vi "Rotate triangle about arbitrary axis.vi"(1 "Rotation angle (rad)":sgl, 2 "Rotation axis coordinates (x, y, z)":sgl[](array[numeric]), 3 "Rotation axis (unit direction vector)\nanti-clockwise positive looking into axis":sgl[](array[numeric]), 4 "Triangle in":T1) -> (0 "Triangle out":T1)   [LabVIEW 2014]
uses:
  Typedefs/Triangle.ctl
panel:
  # "PN 13/01/2015"
  # "Vertices"
  # "Edges"
  # "Unit normal"
  # "pre-store"
  # "Vertices"
  # "Edges"
  # "Unit normal"
  # "pre-store"
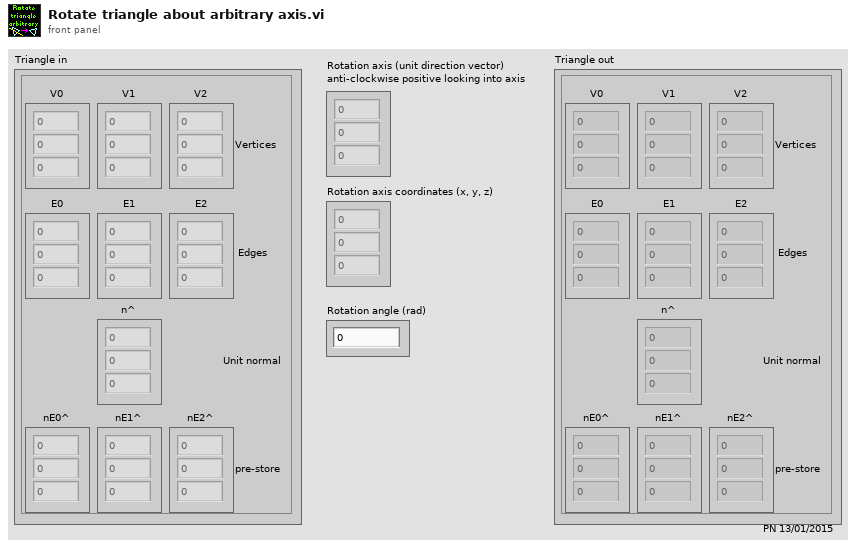
[diagram p1: front panel]
types:
  T1 = typedef "Triangle.ctl" = cluster{"V0":sgl[], "V1":sgl[], "V2":sgl[], "E0":sgl[], "E1":sgl[], "E2":sgl[], "n^":sgl[], "nE0^":sgl[], "nE1^":sgl[], "nE2^":sgl[]}
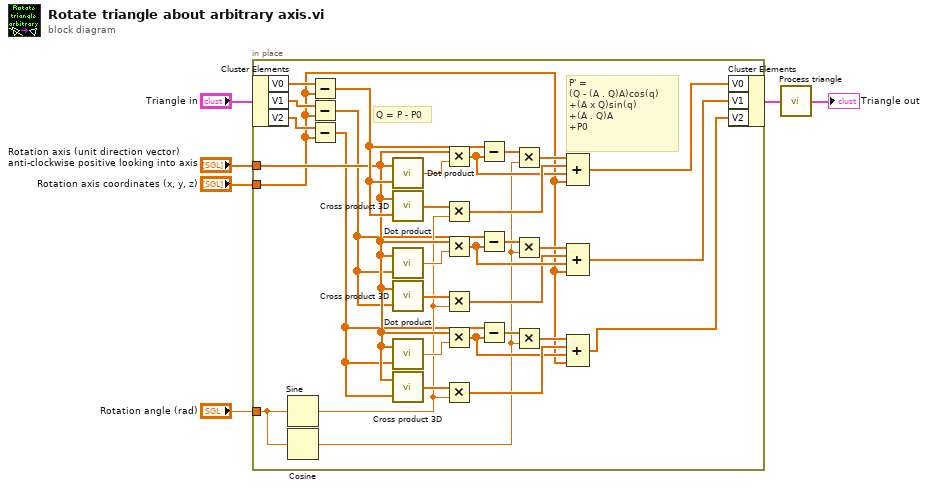
[diagram p0: block diagram]
diagram:
  n1 = in-place {
    in-place-border: "Rotation axis (unit direction vector)\nanti-clockwise positive looking into axis" -> [w13]
    in-place-border: "Rotation axis coordinates (x, y, z)" -> [w12]
    in-place-border: "Rotation angle (rad)" -> [w37]
    # "Q = P - P0"
    # "P' = \n(Q - (A . Q)A)cos(q)\n+(A x Q)sin(q)\n+(A . Q)A\n+P0"
    n2 = in-place-cluster #1("Triangle in") -> ("V0"=w36:sgl[], "V1"=w35:sgl[], "V2"=w34:sgl[])
    n3 = Sine(x=w37) -> (sin(x)=w10:sgl)
    n4 = Cosine(x=w37) -> (cos(x)=w9:sgl)
    n5 = Subtract(x=w36, y=w12) -> (x-y=w14:sgl[])
    n6 = Subtract(x=w35, y=w12) -> (x-y=w8:sgl[])
    n7 = Subtract(x=w34, y=w12) -> (x-y=w7:sgl[])
    n8 = call "Dot product.vi"("B"=w14, "A"=w13) -> ("A . B"=w38:sgl)
    n9 = call "Cross product 3D.vi"("B"=w14, "A"=w13) -> ("A x B"=w32:sgl[])
    n10 = call "Dot product.vi"("B"=w8, "A"=w13) -> ("A . B"=w22:sgl)
    n11 = call "Cross product 3D.vi"("B"=w8, "A"=w13) -> ("A x B"=w24:sgl[])
    n12 = call "Dot product.vi"("B"=w7, "A"=w13) -> ("A . B"=w20:sgl)
    n13 = call "Cross product 3D.vi"("B"=w7, "A"=w13) -> ("A x B"=w18:sgl[])
    n14 = Multiply(x=w13, y=w38) -> (x*y=w29:sgl[])
    n15 = Multiply(x=w32, y=w10) -> (x*y=w30:sgl[])
    n16 = Multiply(x=w13, y=w22) -> (x*y=w27:sgl[])
    n17 = Multiply(x=w24, y=w10) -> (x*y=w26:sgl[])
    n18 = Multiply(x=w13, y=w20) -> (x*y=w15:sgl[])
    n19 = Multiply(x=w18, y=w10) -> (x*y=w16:sgl[])
    n20 = Subtract(x=w14, y=w29) -> (x-y=w33:sgl[])
    n21 = Subtract(x=w8, y=w27) -> (x-y=w23:sgl[])
    n22 = Subtract(x=w7, y=w15) -> (x-y=w19:sgl[])
    n23 = Multiply(x=w33, y=w9) -> (x*y=w31:sgl[])
    n24 = Multiply(x=w23, y=w9) -> (x*y=w25:sgl[])
    n25 = Multiply(x=w19, y=w9) -> (x*y=w17:sgl[])
    n26 = Compound Arithmetic op=ADD(w31, w30, w29, w12) -> (w28:sgl[])
    n27 = Compound Arithmetic op=ADD(w25, w26, w27, w12) -> (w21:sgl[])
    n28 = Compound Arithmetic op=ADD(w17, w16, w15, w12) -> (w11:sgl[])
    n29 = in-place-cluster #1("V0"=w28, "V1"=w21, "V2"=w11) -> (w2:T1)
  }
  n30 = call "Process triangle.vi"("Triangle in"=w2) -> ("Triangle out"=→"Triangle out":T1)
